vi "yellowLocation.vi"() -> (0 "range":string, 1 "pos":string, 2 "Dataout":string="b")   [LabVIEW 2017]
panel:
  out "YELLOW":T1
  out "size":i32
  out "convex hull area":dbl
  out "Tayang":dbl
  out "Area":dbl
  out "Height":dbl
  out "Width":dbl
  out "Bottom":dbl
  out "Right":dbl
  out "Up":dbl
  out "Left":dbl
  out "CenterY":dbl
  out "CenterX":dbl
  out "Yellow_Data":dbl[](array[numeric])
  out "yellow_stop":bool
  out "Numeric":i32
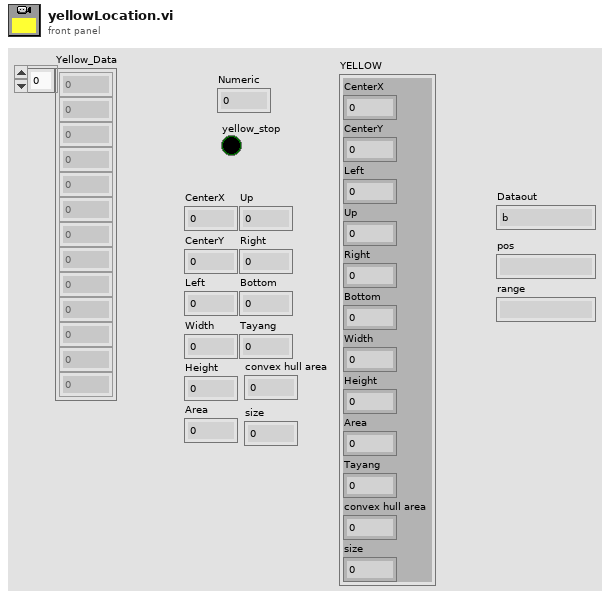
[diagram p1: front panel]
types:
  T1 = cluster{"CenterX":dbl, "CenterY":dbl, "Left":dbl, "Up":dbl, "Right":dbl, "Bottom":dbl, "Width":dbl, "Height":dbl, "Area":dbl, "Tayang":dbl, "convex hull area":dbl, "size":i32}
  T2 = typedef "IMAQ Image.ctl" = refnum<image>
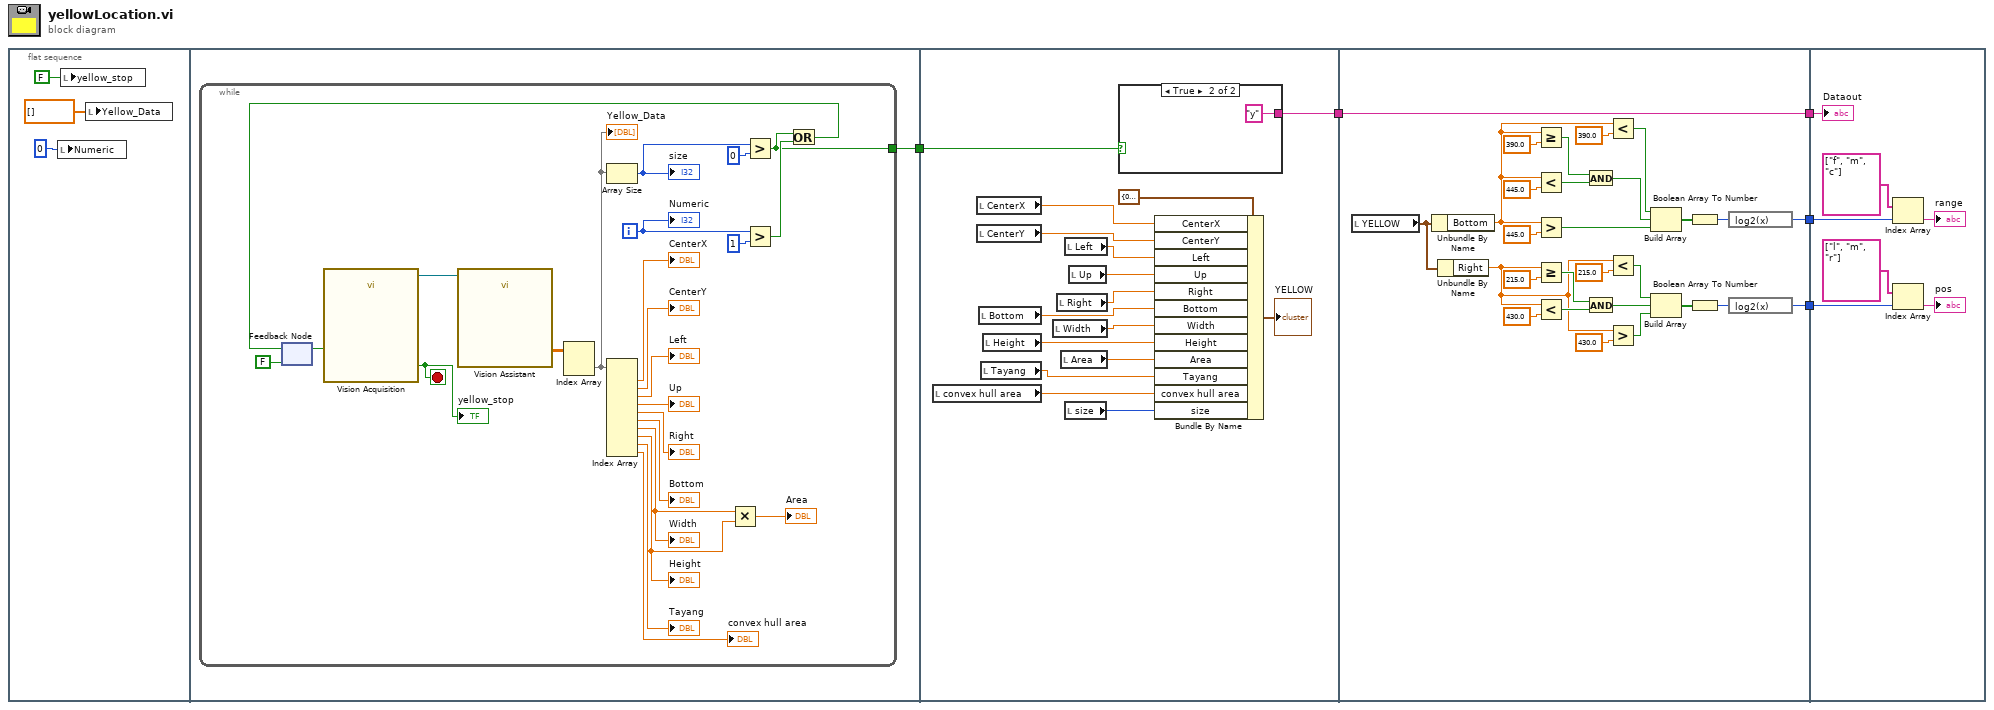
[diagram p0: block diagram]
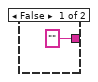
[diagram p2: hidden frame]
diagram:
  n1 = flat-sequence {
    tunnel: [w9] -> w5
    tunnel: w5 -> [w35]
    tunnel: [w34] -> w3
    tunnel: [w79] -> w4
    tunnel: w3 -> [w79]
    tunnel: [w53] -> w2
    tunnel: [w52] -> w1
    tunnel: w4 -> [w86]
    tunnel: w2 -> [w81]
    tunnel: w1 -> [w80]
    frame #0 {
      n2 = local write "Numeric"(0 ("Numeric")) -> ()
      n3 = local write "yellow_stop"(FALSE ("yellow_stop")) -> ()
      n4 = local write "Yellow_Data"(dbl[] [] ("Yellow_Data")) -> ()
    }
    frame #1 {
      n5 = while {
        tunnel: [w10] -> w9
        i -> [w28]
        stop <- w23 stop-if-true
        n6 = feedback #1(FALSE) -> (w25:bool)
        n7 = call "Vision Acquisition"("Stop (F)"=w25) -> ("Image Out"=w33:T2, "Stopped"=w23:bool)  [unwired: 24 in, 1 out]
        "yellow_stop" <- w23
        n8 = call "Vision Assistant"("Image In"=w33) -> ("Particle Measurements (Pixels) (Particle Analysis 1)"=w32:dbl[][])  [unwired: 23 in, 3 out]
        n9 = Index Array(array=w32) -> (element=w11:dbl[])  [unwired: 2 in]
        "Yellow_Data" <- w11
        n10 = Array Size(array=w11) -> (size(s)=w31:i32)
        "size" <- w31
        n11 = Index Array(array=w11) -> (element #1=→"CenterX":dbl, element #2=→"CenterY":dbl, element #3=→"Left":dbl, element #4=→"Up":dbl, element #5=→"Right":dbl, element #6=→"Bottom":dbl, element #7=w22:dbl, element #8=w21:dbl, element #9=→"Tayang":dbl, element #10=→"convex hull area":dbl)  [unwired: 10 in]
        "Width" <- w22
        "Height" <- w21
        n12 = Multiply(x=w22, y=w21) -> (x*y=→"Area":dbl)
        n13 = Greater?(x=w31, y=0) -> (0:w10:bool)
        n14 = Greater?(x=w28, y=1) -> (0:w27:bool)
        n15 = Or(x=w10, y=w27) -> (x .or. y?=w26:bool)
        n16 = feedback-in #1(w26) -> ()
        "Numeric" <- w28
      }
    }
    frame #2 {
      n17 = local read "convex hull area"() -> (w39:dbl)
      n18 = local read "CenterX"() -> (w49:dbl)
      n19 = local read "CenterY"() -> (w48:dbl)
      n20 = local read "Bottom"() -> (w44:dbl)
      n21 = local read "Tayang"() -> (w40:dbl)
      n22 = local read "Height"() -> (w42:dbl)
      n23 = local read "Width"() -> (w43:dbl)
      n24 = local read "Right"() -> (w45:dbl)
      n25 = local read "Area"() -> (w41:dbl)
      n26 = local read "Left"() -> (w47:dbl)
      n27 = local read "size"() -> (w38:i32)
      n28 = local read "Up"() -> (w46:dbl)
      n29 = case shown="True" w35 {
        tunnel: ["" "y"] -> w34
        frame False {
        }
        frame True {
        }
      }
      n30 = Bundle By Name(cluster=T1 {"CenterX"=0.0, "CenterY"=0.0, "Left"=0.0, "Up"=0.0, "Right"=0.0, "Bottom"=0.0, "Width"=0.0, "Height"=0.0, "Area"=0.0, "Tayang"=0.0, "convex hull area"=0.0, "size"=0} ("output cluster"), "CenterX"=w49, "CenterY"=w48, "Left"=w47, "Up"=w46, "Right"=w45, "Bottom"=w44, "Width"=w43, "Height"=w42, "Area"=w41, "Tayang"=w40, "convex hull area"=w39, "size"=w38) -> (→"YELLOW":T1)
    }
    frame #3 {
      n31 = local read "YELLOW"() -> (w54:T1)
      n32 = Unbundle By Name(w54) -> ("Bottom"=w56:dbl)
      n33 = Unbundle By Name(w54) -> ("Right"=w55:dbl)
      n34 = Greater Or Equal?(x=w56, y=390.0) -> (x >= y?=w64:bool)
      n35 = Less?(x=w56, y=445.0) -> (x < y?=w63:bool)
      n36 = Greater?(x=w56, y=445.0) -> (0:w57:bool)
      n37 = Greater Or Equal?(x=w55, y=215.0) -> (x >= y?=w75:bool)
      n38 = Less?(x=w55, y=430.0) -> (x < y?=w74:bool)
      n39 = And(x=w64, y=w63) -> (x .and. y?=w58:bool)
      n40 = And(x=w75, y=w74) -> (x .and. y?=w71:bool)
      n41 = Less?(x=w56, y=390.0) -> (x < y?=w59:bool)
      n42 = Less?(x=w55, y=215.0) -> (x < y?=w72:bool)
      n43 = Greater?(x=w55, y=430.0) -> (0:w70:bool)
      n44 = Build Array(w59, w58, w57) -> (w61:bool[])
      n45 = Build Array(w72, w71, w70) -> (w69:bool[])
      n46 = Boolean Array To Number(Boolean array=w61) -> (number=w60:u32)
      n47 = Boolean Array To Number(Boolean array=w69) -> (number=w68:u32)
      n48 = expression code="log2(x)"(w60) -> (w52:u32)
      n49 = expression code="log2(x)"(w68) -> (w53:u32)
    }
    frame #4 {
      n50 = Index Array(array=string[] ["f", "m", "c"], index=w80) -> (element=→"range":string)
      n51 = Index Array(array=string[] ["l", "m", "r"], index=w81) -> (element=→"pos":string)
      "Dataout" <- w86
    }
  }
